vi "Empty.vi"(8 "error in (no error)":errorcluster, 11 "Client in":T1) -> (0 "error out":errorcluster, 3 "Client out":T1)   [LabVIEW 2013, in "Client.lvlib" / "Client.lvclass"]
doc: "Vi with an error case structure and object reference I/O. Can be copied as a starting point for new function implementations."
uses:
  Client.lvclass
  Object-reference.ctl
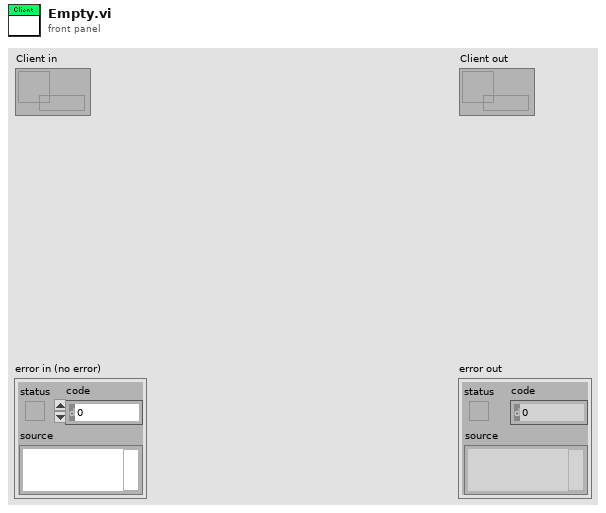
[diagram p1: front panel]
types:
  T1 = typedef "Client.lvlib/Client.lvclass/Object-reference.ctl" = refnum<data-value>
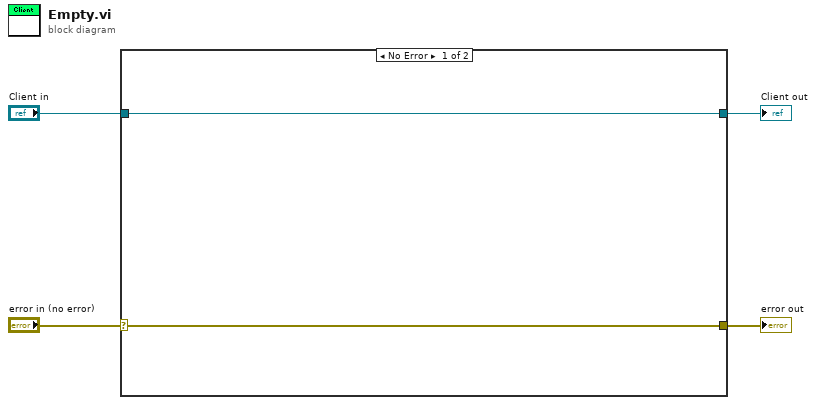
[diagram p0: block diagram]
diagram:
  n1 = case shown="No Error" "error in (no error)" {
    selector: "error in (no error)" -> [w6 w8]
    tunnel: [w6 w8] -> w3
    tunnel: [w5 w7] -> w1
    tunnel: "Client in" -> [w5 w7]
    frame No Error {
    }
    frame Error {
    }
  }
  "error out" <- w3
  "Client out" <- w1
